vi "line to strings.vi"(11 "line":T1) -> (3 "strings":string[](array[string]))   [LabVIEW 2013, in "Modbus Slave editor node.lvclass"]
doc: "Platypus Framework 1.0.1.65\nNI Systems Engineering - National Instruments"
uses:
  Modbus Slave editor node.lvclass
  table line.ctl
  <vilib>/NI/TBM Modules/modbus slave/module channel/Modbus Module Channel.lvclass
  <vilib>/NI/Tag Bus/tag/tag descriptor.lvclass/tag descriptor.ctl
  <vilib>/NI/TBM Modules/modbus slave/module channel/Modbus Module Channel.lvclass/Modbus Module Channel.ctl
  <vilib>/NI/Tag Bus Module Framework/channel/TBM channel.lvclass/TBM channel.ctl
  <vilib>/NI/Tag Bus/tag/read tag name.vi
  <vilib>/NI/TBM Modules/modbus slave/module channel/Read modbus type.vi
  <vilib>/NI/TBM Modules/modbus slave/module channel/Read starting address.vi
  <vilib>/NI/TBM Modules/modbus slave/module channel/Read subindex (bool).vi
  <vilib>/NI/Tag Bus Module Framework/channel/Read channel classification.vi
  <vilib>/NI/Tag Bus/tag/read data type.vi
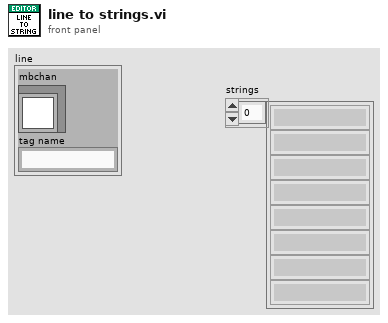
[diagram p1: front panel]
types:
  T1 = typedef "Modbus Slave editor node.lvclass/table line.ctl" = cluster{"mbchan":refnum<class "Modbus Module Channel.lvclass">, "tag name":string}
  T2 = typedef "Modbus Module Channel.lvclass/data bank type.ctl" = enum16{"coils", "discrete inputs", "input registers", "holding registers"}
  T3 = typedef "TBM channel.lvclass/channel classification.ctl" = enum16{"input data", "output data", "processing parameter", "processing result"}
  T4 = typedef "tag bus.lvlib/tag descriptor.lvclass/Data Type.ctl" = enum16{"Double", "Single", "I64", "I32", "I16", "I8", "U64", "U32", "U16", "U8", "Boolean", "String", "Array of Double", "Array of Single", "Array of I64", "Array of I32", "Array of I16", "Array of I8", "Array of U64", "Array of U32", "Array of U16", "Array of U8", "Array of Boolean", "Array of String"}
  T5 = typedef "Modbus Slave editor node.lvclass/permissions.ctl" = enum32{"Read from MB", "Write to MB"}
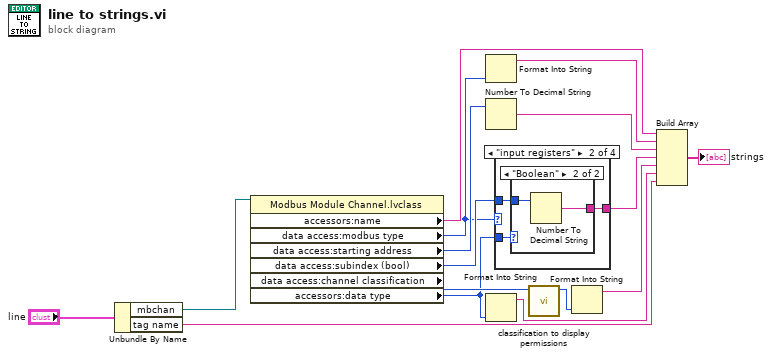
[diagram p0: block diagram]
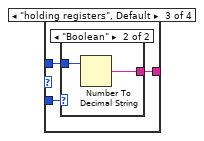
[diagram p4: hidden frame]
diagram:
  n1 = Unbundle By Name("line") -> ("mbchan"=w10:refnum<class "Modbus Module Channel.lvclass">, "tag name"=w14:string)
  n2 = property class="Modbus Module Channel.lvclass"(reference=w10) -> ("accessors:name"=w8:string, "data access:modbus type"=w1:T2, "data access:starting address"=w4:u16, "data access:subindex (bool)"=w7:i32, "data access:channel classification"=w9:T3, "accessors:data type"=w5:T4)  [unwired: 1 in, 2 out]
  n3 = Format Into String(w1) -> (resulting string=w2:string)  [unwired: 3 in, 1 out]
  n4 = Number To Decimal String(number=w4) -> (decimal integer string=w3:string)  [unwired: 1 in]
  n5 = Format Into String(w5) -> (resulting string=w15:string)  [unwired: 3 in, 1 out]
  n6 = case shown="\"input registers\"" w1 {
    tunnel: w7 -> [_ w19 w24 _]
    tunnel: [_ w18 w23 _] -> w6
    tunnel: w5 -> [_ w17 w22 _]
    frame "discrete inputs" {
    }
    frame "input registers" {
      n7 = case shown="\"Boolean\"" w17 {
        tunnel: w19 -> [_ w21]
        tunnel: [_ w20] -> w18
        frame "Double", Default {
        }
        frame "Boolean" {
          n8 = Number To Decimal String(number=w21) -> (decimal integer string=w20:string)  [unwired: 1 in]
        }
      }
    }
    frame "holding registers", Default {
      n9 = case shown="\"Boolean\"" w22 {
        tunnel: w24 -> [_ w26]
        tunnel: [_ w25] -> w23
        frame "Double", Default {
        }
        frame "Boolean" {
          n10 = Number To Decimal String(number=w26) -> (decimal integer string=w25:string)  [unwired: 1 in]
        }
      }
    }
    frame "coils" {
    }
  }
  n11 = call "classification to display permissions.vi"("channel classification"=w9) -> ("permissions"=w12:T5)  [unwired: 10 in]
  n12 = Format Into String(w12) -> (resulting string=w11:string)  [unwired: 3 in, 1 out]
  n13 = Build Array(w8, w2, w3, w6, w11, w15, w14) -> (→"strings":string[])
